vi "Print.vi"(8 "error in":errorcluster, 10 "Anything In":variant, 11 "JSON Printer in":refnum<class "JSON Printer.lvclass">) -> (0 "error out":errorcluster, 2 "Printed String":string, 3 "JSON Printer out":refnum<class "JSON Printer.lvclass">)   [LabVIEW 2020, in "Approval Tests.lvlib" / "JSON Printer.lvclass"]
uses:
  JSON Printer.lvclass
  <vilib>/PNR/JSONtext Object Serialization/Generic Object Serializer/Generic Object Serializer.lvclass
  C:/Program Files/National Instruments/LabVIEW 2020/vi.lib/JDP Science/JSONtext/LVClass Serializer/JSONtext LVClass Serializer.lvclass
  35ec3b54-d4f0-4625-b2e1-f9ec705186b8.vi
  <vilib>/JDP Science/JSONtext/Variant to JSON Text.vi
  JSON Printer.lvclass/JSON Printer.ctl
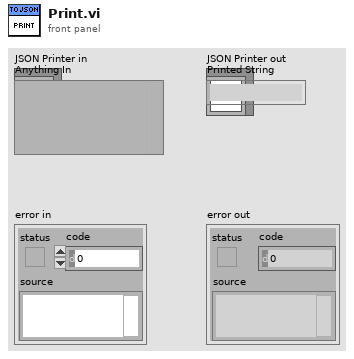
[diagram p1: front panel]
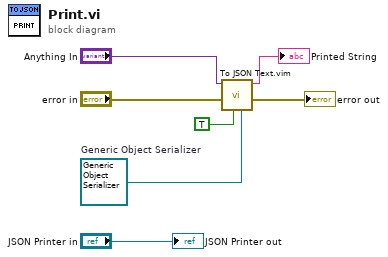
[diagram p0: block diagram]
diagram:
  w3 = refnum<class "Generic Object Serializer.lvclass"> refnum  # Generic Object Serializer
  n1 = call "To JSON Text.vim"("LVClass Serializer"=w3, "Pretty Print?"=TRUE, "error in (no error)"="error in", "Anything"="Anything In") -> ("error out"=→"error out":errorcluster, "<JSON>"=→"Printed String":string)  [unwired: 6 in]
  "JSON Printer out" <- "JSON Printer in"
